vi "RemoveNode.vi"(8 "error in":errorcluster, 10 "node":T1) -> (0 "error out":errorcluster, 2 "node ID":string)   [LabVIEW 2013, in "NISE_CEF_TreeControl.lvlib"]
doc: "Removes the node , deleting all the references to it and destroying the references"
uses:
  NISE_CEF_TreeControl.lvlib
  Node/NodeRef.ctl
  Node/NISE_CEF_Node.lvclass
  Node/NISE_CEF_Node.lvclass/NISE_CEF_Node.ctl
  Node/ReadParent.vi
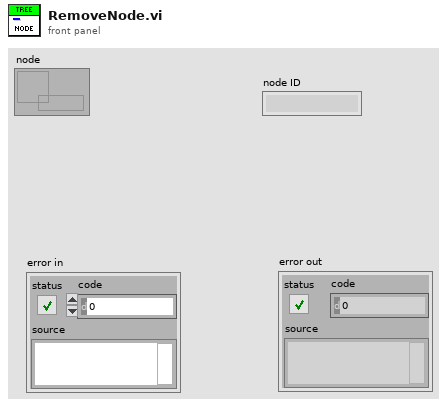
[diagram p1: front panel]
types:
  T1 = typedef "NISE_CEF_Node.lvclass/NodeRef.ctl" = refnum<data-value>
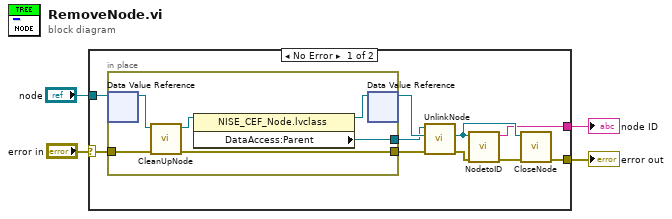
[diagram p0: block diagram]
diagram:
  n1 = case shown="No Error" "error in" {
    selector: "error in" -> [w6 w21]
    tunnel: [w8 w21] -> w3
    tunnel: "node" -> [w14 _]
    tunnel: [w7 _] -> w1
    frame No Error {
      n2 = in-place {
        in-place-border: [w19] -> w12
        in-place-border: w6 -> [w16]
        in-place-border: [w15] -> w5
        n3 = in-place-dvr #1(w14) -> (w18:refnum<class "NISE_CEF_Node.lvclass">)  [unwired: 1 out]
        n4 = call-dynamic "CleanUpNode.vi"("error in (no error)"=w16, "NISE_CEF_Node in"=w18) -> ("error out"=w15:errorcluster, "NISE_CEF_Node out"=w17:refnum<class "NISE_CEF_Node.lvclass">)  [unwired: 8 in]
        n5 = property class="NISE_CEF_Node.lvclass"(reference=w17) -> (reference out=w20:refnum<class "NISE_CEF_Node.lvclass">, "DataAccess:Parent"=w19:T1)  [unwired: 1 in, 1 out]
        n6 = in-place-dvr #1(w20) -> (w13:T1)  [unwired: 1 out]
      }
      n7 = call "UnlinkNode.vi"("error in"=w5, "child in"=w13, "parent in"=w12) -> ("error out"=w9:errorcluster, "child out"=w10:T1)  [unwired: 6 in, 1 out]
      n8 = call "NodetoID.vi"("error in"=w9, "node ref"=w10) -> ("error out"=w11:errorcluster, "ID"=w7:string)  [unwired: 8 in]
      n9 = call "CloseNode.vi"("error in"=w11, "node ref"=w10) -> ("error out"=w8:errorcluster)  [unwired: 9 in]
    }
    frame Error {
    }
  }
  "error out" <- w3
  "node ID" <- w1
